vi "Remove Zeroes.vi"(8 "error in (no error)":errorcluster, 11 "Sensor Information in":T1) -> (0 "error out":errorcluster, 3 "Sensor Information out":T1)   [LabVIEW 2026]
uses:
  controls/Messaging Payloads/Sensor CoreData.ctl
  controls/Messaging Payloads/Sensor CoreData Cluster.ctl
  controls/UI/Units Enum.ctl
  controls/UI/Signal Enum.ctl
  Settings/Settings.lvlib
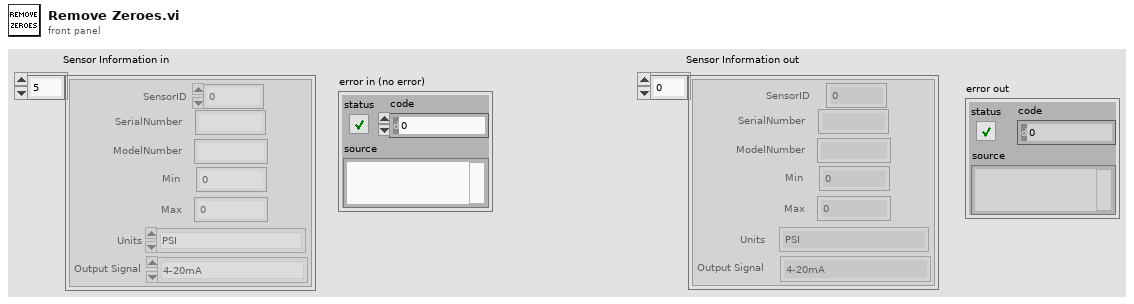
[diagram p1: front panel]
types:
  T1 = typedef "Sensor CoreData.ctl" = T2[]
  T2 = typedef "Settings.lvlib/Sensor CoreData Cluster.ctl" = cluster{"SerialNumber":string, "ModelNumber":string, "Min":dbl, "Max":dbl, "Units":T3, "Output Signal":T4, "SensorID":i32}
  T3 = typedef "Units Enum.ctl" = enum16{"PSI", "Deg C", "kPa", "GPM"}
  T4 = typedef "Signal Enum.ctl" = enum16{"4-20mA", "0-10V", "Thermocouple Type K"}
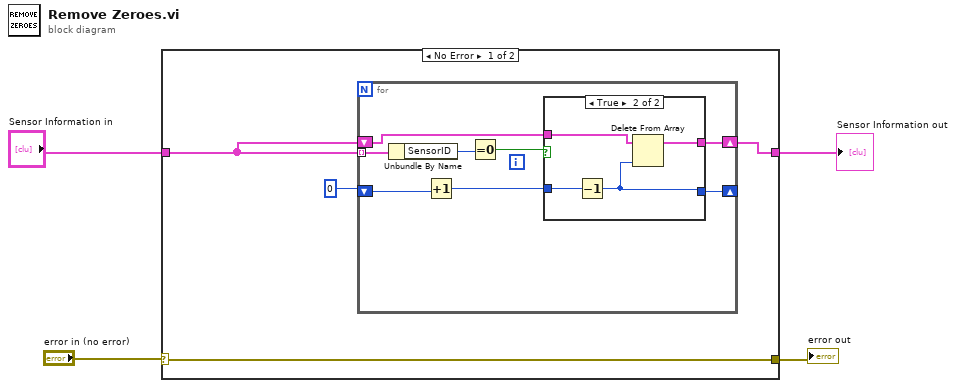
[diagram p0: block diagram]
diagram:
  n1 = case shown="No Error" "error in (no error)" {
    selector: "error in (no error)" -> [w6 w24]
    tunnel: "Sensor Information in" -> [w8 w23]
    tunnel: [w7 w23] -> w1
    tunnel: [w6 w24] -> w3
    frame No Error {
      n2 = for {
        tunnel: w8 -> [w16] mode=indexing
        shift-right: [w12] -> w7
        shift-left: w8 -> [w13]
        shift-right: [w11] -> _
        shift-left: 0 -> [w10]
        n3 = Unbundle By Name(w16) -> ("SensorID"=w15:i32)
        n4 = Increment(x=w10) -> (x+1=w9:i32)
        n5 = Equal To 0?(x=w15) -> (x = 0?=w14:bool)
        n6 = case shown="True" w14 {
          tunnel: w13 -> [w18 w22]
          tunnel: [w18 w21] -> w12
          tunnel: [w17 w19] -> w11
          tunnel: w9 -> [w17 w20]
          frame False {
          }
          frame True {
            n7 = Decrement(x=w20) -> (x-1=w19:i32)
            n8 = Delete From Array(array=w22, index=w19) -> (array with subset deleted=w21:T1)  [unwired: 1 in, 1 out]
          }
        }
      }
    }
    frame Error {
    }
  }
  "error out" <- w3
  "Sensor Information out" <- w1
